vi "UpdateHistory.vi"(8 "error in (no error)":errorcluster, 10 "Json Data":string, 11 "WebSocket in":refnum<class "WebSocket.lvclass">) -> (0 "error out":errorcluster, 3 "WebSocket out":refnum<class "WebSocket.lvclass">)   [LabVIEW 2019, in "WebSocket.lvlib" / "WebSocket.lvclass"]
uses:
  WebSocket.lvclass
  Models/ImageResultModel.ctl
  074d6f64-3082-4cef-823e-993c6beebb41.vi
  c45f76cb-1895-4486-b71c-b00d899104c4.vi
  <vilib>/JDP Science/JSONtext/JSON text to Variant.vi
  <vilib>/JDP Science/JSONtext/Variant to JSON Text.vi
  <vilib>/JDP Science/JSONtext/LVClass Serializer/JSONtext LVClass Serializer.lvclass
panel:
  out "x-y":u32
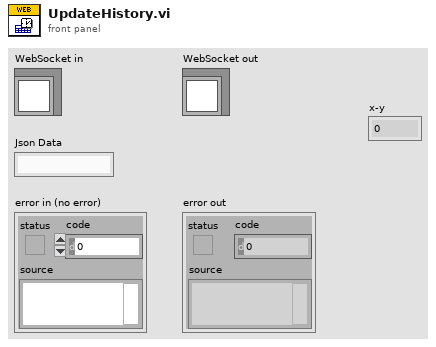
[diagram p1: front panel]
types:
  T1 = typedef "ImageResultModel.ctl" = cluster{"image":string, "pass":bool, "class":string, "time":dbl}
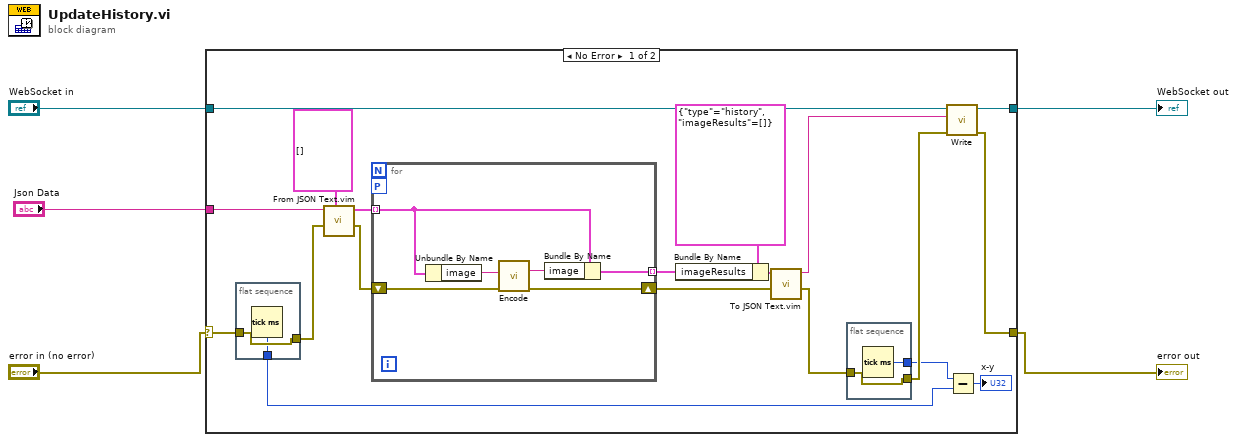
[diagram p0: block diagram]
diagram:
  n1 = case shown="No Error" "error in (no error)" {
    selector: "error in (no error)" -> [w18 w36]
    tunnel: [w22 w36] -> w1
    tunnel: [w21 w35] -> w2
    tunnel: "WebSocket in" -> [w23 w35]
    tunnel: "Json Data" -> [w20 _]
    frame No Error {
      n2 = flat-sequence {
        tunnel: w18 -> [w34]
        tunnel: [w34] -> w17
        tunnel: [w33] -> w14
        frame #0 {
          n3 = Tick Count (ms)() -> (millisecond timer value=w33:u32)
        }
      }
      n4 = call "From JSON Text.vim"("Data Type and Default Value"=T1[] [] ("Array"), "error in (no error)"=w17, "JSON"=w20) -> ("error out"=w19:errorcluster, "Data out"=w11:T1[])  [unwired: 7 in]
      n5 = for {
        tunnel: w11 -> [w29] mode=indexing
        shift-right: [w26] -> w9
        shift-left: w19 -> [w30]
        workers-P: _ -> [_]
        tunnel: [w25] -> w6 mode=indexing
        n6 = Unbundle By Name(w29) -> ("image"=w28:string)
        n7 = call "Encode.vi"("error in (no error)"=w30, "string in (not encoded)"=w28) -> ("error out"=w26:errorcluster, "string out (base64-encoded)"=w27:string)  [unwired: 8 in]
        n8 = Bundle By Name(cluster=w29, "image"=w27) -> (w25:T1)
      }
      n9 = Bundle By Name(cluster=cluster{"type":string, "imageResults":T1[]} {"type"="history", "imageResults"=[]}, "imageResults"=w6) -> (w10:cluster{"type":string, "imageResults":T1[]})
      n10 = call "To JSON Text.vim"("error in (no error)"=w9, "Anything"=w10) -> ("error out"=w8:errorcluster, "<JSON>"=w7:string)  [unwired: 8 in]
      n11 = flat-sequence {
        tunnel: w8 -> [w32]
        tunnel: [w32] -> w16
        tunnel: [w31] -> w15
        frame #0 {
          n12 = Tick Count (ms)() -> (millisecond timer value=w31:u32)
        }
      }
      n13 = call "Write.vi"("error in (no error)"=w16, "Write"=w7, "WebSocket in"=w23) -> ("error out"=w22:errorcluster, "WebSocket out"=w21:refnum<class "WebSocket.lvclass">)  [unwired: 7 in]
      n14 = Subtract(x=w15, y=w14) -> (x-y=→"x-y":u32)
    }
    frame Error {
    }
  }
  "error out" <- w1
  "WebSocket out" <- w2
